vi "IMS Stepper Init.vi"(2 "error in (no error)":errorcluster, 3 "Baud Rate":u32=9600, 4 "Motor Number":u32=1 min=1 max=255 step=1, 5 "Instrument Address":refnum<visa-resource-name>) -> (0 "error out":errorcluster, 1 "Response":string)   [LabVIEW 2019]
uses:
  Serial Support VISA.llb/Serial Actions.ctl
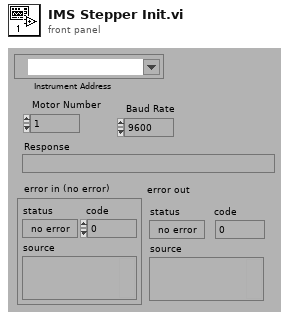
[diagram p1: front panel]
types:
  T1 = cluster{"flow control":enum16{"None", "XON/XOFF", "RTS/CTS"}, "baud rate":u32, "data bits":u16, "Stop Bits":u16, "parity (0:none)":enum16{"None", "Odd", "Even", "Mark", "Space"}, "Transmit Buffer Size":u32, "Receive Buffer Size":u32}
  T2 = typedef "Serial Actions.ctl" = enum16{"Init", "Break", "Clear Buffer", "Write", "Read", "N Bytes", "Lock", "Unlock", "Close"}
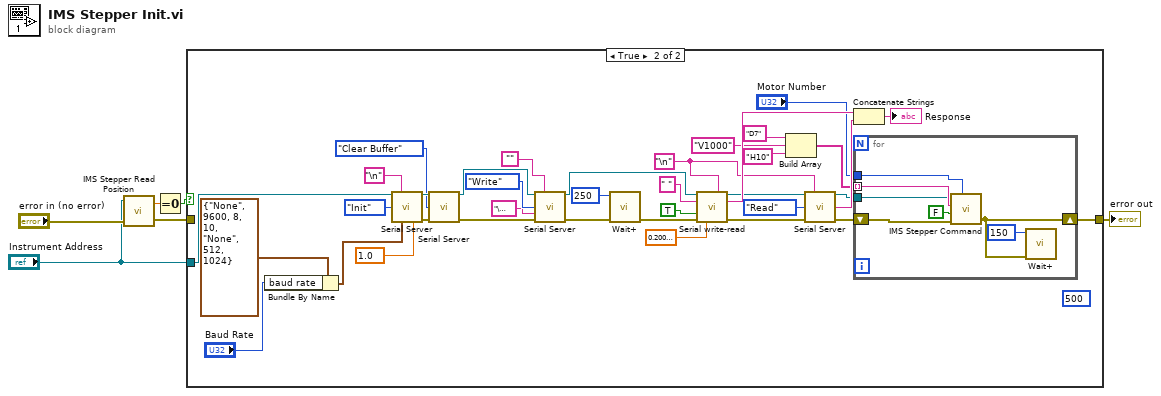
[diagram p0: block diagram]
diagram:
  n1 = call "IMS Stepper Read Position.vi"("error in (no error)"="error in (no error)", "Instrument Address"="Instrument Address") -> ("error out"=w6:errorcluster, "Response"=w1:dbl)  [unwired: 1 in]
  n2 = Equal To 0?(x=w1) -> (x = 0?=w2:bool)
  n3 = case shown="True" w2 {
    tunnel: w6 -> [w7 _]
    tunnel: "Instrument Address" -> [_ w10]
    tunnel: [w7 w9] -> w3
    frame False {
    }
    frame True {
      w27 = "\n" ("EOT Chars (cr/lf)")
      (unwired) u32 500 ("Max Char to Read")
      n4 = Bundle By Name(cluster=T1 {"flow control"=enum."None", "baud rate"=9600, "data bits"=8, "Stop Bits"=10, "parity (0:none)"=enum."None", "Transmit Buffer Size"=512, "Receive Buffer Size"=1024} ("Port Parameters"), "baud rate"="Baud Rate") -> (w20:T1)
      n5 = call "Serial Server.vi"("VISA Resource Name"=w10, "EOT Chars (cr/lf)"="\n", "Action"=Serial_Actions."Init", "Port Parameters"=w20, "Timeout Limit(sec)"=1.0 ("Timeout Limit")) -> ("dup VISA Resource Name"=w19:refnum<visa-resource-name>, "error out"=w16:errorcluster)  [unwired: 6 in, 3 out]
      n6 = call "Serial Server.vi"("VISA Resource Name"=w19, "Action"=Serial_Actions."Clear Buffer", "error in (no error)"=w16) -> ("dup VISA Resource Name"=w43:refnum<visa-resource-name>, "error out"=w42:errorcluster)  [unwired: 8 in, 3 out]
      n7 = call "Serial Server.vi"("VISA Resource Name"=w43, "EOT Chars (cr/lf)"="", "Action"=Serial_Actions."Write", "String To Send"="\u0003" ("Command"), "error in (no error)"=w42) -> ("dup VISA Resource Name"=w44:refnum<visa-resource-name>, "error out"=w37:errorcluster)  [unwired: 6 in, 3 out]
      n8 = call "Wait+.vi"("Error In"=w37, "milliseconds to wait"=u32 250) -> ("Error Out"=w41:errorcluster)  [unwired: 4 in, 1 out]
      n9 = call "Serial write-read.vi"("VISA Resource Name"=w44, "EOT Chars (cr/lf)"=w27, "String To Send"=" " ("Command"), "Clear Buffer?"=TRUE, "error in (no error)"=w41, "Timeout Limit"=sgl 0.2) -> ("dup VISA Resource Name"=w31:refnum<visa-resource-name>, "Serial Read"=w33:string, "error out"=w32:errorcluster)  [unwired: 4 in, 3 out]
      n10 = Build Array("D7", "V1000", "H10") -> (w12:string[])
      n11 = call "Serial Server.vi"("VISA Resource Name"=w31, "EOT Chars (cr/lf)"=w27, "Action"=Serial_Actions."Read", "error in (no error)"=w32) -> ("dup VISA Resource Name"=w29:refnum<visa-resource-name>, "Serial Read"=w35:string, "error out"=w28:errorcluster)  [unwired: 7 in, 2 out]
      n12 = Concatenate Strings(w33, w35) -> (→"Response":string)
      n13 = for {
        shift-right: [w46] -> w9
        shift-left: w28 -> [w47]
        tunnel: w12 -> [w50] mode=indexing
        tunnel: "Motor Number" -> [w49]
        tunnel: w29 -> [w48]
        n14 = call "IMS Stepper Command.vi"("Instrument Address"=w48, "Motor Number"=w49, "Command"=w50, "Mode"=FALSE, "error in (no error)"=w47) -> ("error out"=w46:errorcluster)  [unwired: 1 in, 2 out]
        n15 = call "Wait+.vi"("Error In"=w46, "milliseconds to wait"=u32 150) -> ()  [unwired: 4 in, 2 out]
      }
    }
  }
  "error out" <- w3
